vi "analogmultiple.vi"() -> ()   [LabVIEW 2022 SP3]
uses:
  <vilib>/DAQmx/read.llb/DAQmx Read (Analog 2D DBL NChan NSamp).vi
  <vilib>/DAQmx/create/channels.llb/DAQmx Create Channel (AI-Voltage-Basic).vi
  <vilib>/DAQmx/miscellaneous.llb/DAQmx Fill In Error Info.vi
panel:
  in  "physical channels 3":tag
  out "Waveform Chart":dbl[](graph)
  in  "stop":bool
  out "Waveform Chart 2":dbl[](graph)
  in  "physical channels":tag
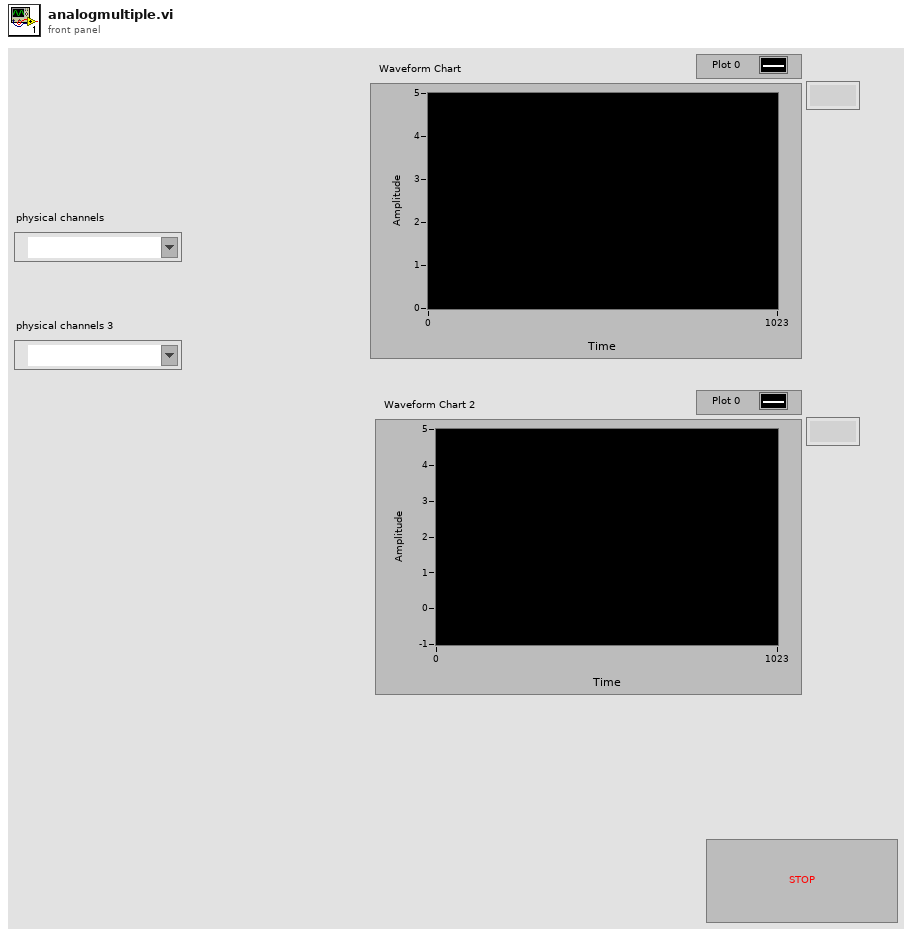
[diagram p1: front panel]
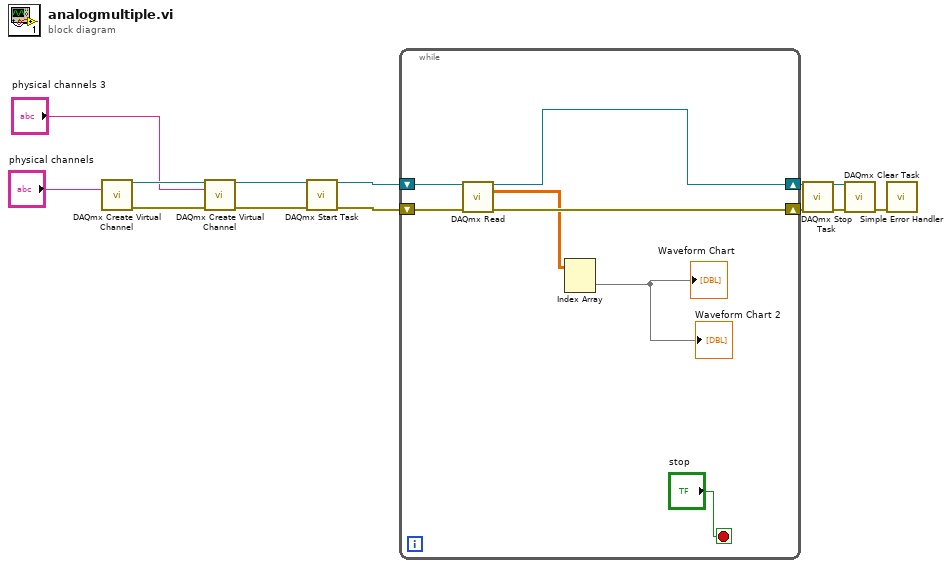
[diagram p0: block diagram]
diagram:
  n1 = call-poly <vilib>:"DAQmx Create Virtual Channel.vi"("physical channels"="physical channels") -> ("task out"=w5:refnum<k21>, "error out"=w2:errorcluster)  [unwired: 13 in]
  n2 = call-poly <vilib>:"DAQmx Create Virtual Channel.vi"("task in"=w5, "physical channels"="physical channels 3", "error in"=w2) -> ("task out"=w4:refnum<k21>, "error out"=w1:errorcluster)  [unwired: 11 in]
  n3 = call <vilib>:"DAQmx Start Task.vi"("task/channels in"=w4, "error in"=w1) -> ("task out"=w13:refnum<k21>, "error out"=w9:errorcluster)  [unwired: 12 in]
  n4 = while {
    shift-right: [w19] -> w12
    shift-left: w13 -> [w20]
    shift-right: [w17] -> w8
    shift-left: w9 -> [w18]
    stop <- "stop" stop-if-true
    n5 = call-poly <vilib>:"DAQmx Read.vi"("task/channels in"=w20, "error in"=w18) -> ("task out"=w19:refnum<k21>, "data"=w15:dbl[][], "error out"=w17:errorcluster)  [unwired: 11 in]
    n6 = Index Array(array=w15) -> (element=→"Waveform Chart" →"Waveform Chart 2":dbl[])  [unwired: 2 in]
  }
  n7 = call <vilib>:"DAQmx Stop Task.vi"("task/channels in"=w12, "error in"=w8) -> ("task out"=w11:refnum<k21>, "error out"=w7:errorcluster)  [unwired: 12 in]
  n8 = call <vilib>:"DAQmx Clear Task.vi"("task in"=w11, "error in"=w7) -> ("error out"=w10:errorcluster)  [unwired: 13 in]
  n9 = call <vilib>:"Simple Error Handler.vi"("error in (no error)"=w10) -> ()  [unwired: 4 in, 5 out]
